vi "Write Data Raw reference.vi"(8 "error in (no error)":errorcluster, 11 "DATA in":refnum<class "DATA.lvclass">) -> (0 "error out":errorcluster, 3 "DATA out":refnum<class "DATA.lvclass">)   [LabVIEW 2018, in "DATA.lvclass"]
uses:
  DATA.lvclass
  DATA.lvclass/DATA.ctl
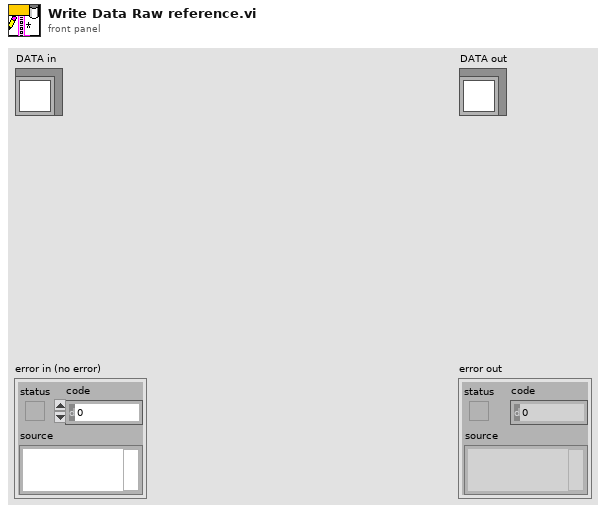
[diagram p1: front panel]
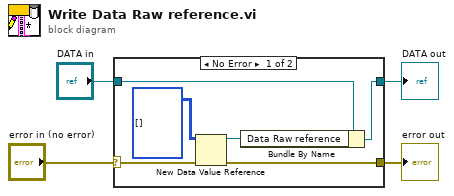
[diagram p0: block diagram]
diagram:
  n1 = case shown="No Error" "error in (no error)" {
    selector: "error in (no error)" -> [w6 w11]
    tunnel: [w5 w11] -> w3
    tunnel: [w9 w12] -> w1
    tunnel: "DATA in" -> [w10 w12]
    frame No Error {
      n2 = New Data Value Reference(data value=i32[][][][] [], error in=w6) -> (data value reference=w7:refnum<data-value>, error out=w5:errorcluster)
      n3 = Bundle By Name(cluster=w10, "Data Raw reference"=w7) -> (w9:refnum<class "DATA.lvclass">)
    }
    frame Error {
    }
  }
  "error out" <- w3
  "DATA out" <- w1
